vi "DSF.Shared.Configuration.Framework.Get Path.vi"(11 "Framework Configuration in":refnum<class "DSF.Shared.Configuration.Framework.lvclass">) -> (2 "configuration path":path, 3 "Framework Configuration out":refnum<class "DSF.Shared.Configuration.Framework.lvclass">)   [LabVIEW 2017, in "DSF.Engine.lvlib" / "DSF.Shared.Configuration.Framework.lvclass"]
uses:
  DSF.Shared.Configuration.Framework.lvclass
  DSF.Shared.Configuration.Framework.lvclass/DSF.Shared.Configuration.Framework.ctl
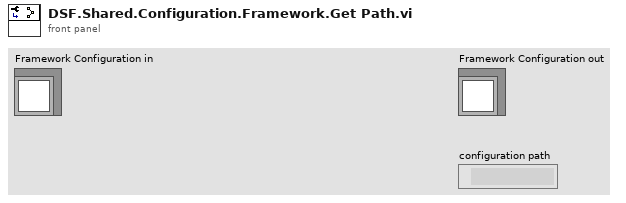
[diagram p1: front panel]
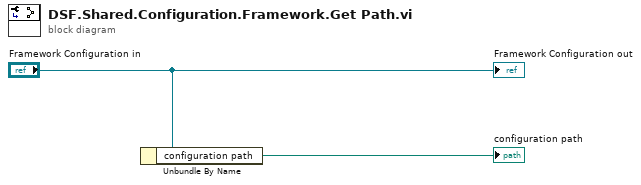
[diagram p0: block diagram]
diagram:
  n1 = Unbundle By Name("Framework Configuration in") -> ("configuration path"=→"configuration path":path)
  "Framework Configuration out" <- "Framework Configuration in"
